vi "OutFlagJudge.vi"(8 "error in":errorcluster caption="错误输入", 11 "包装箱条码":string) -> (0 "error out":errorcluster caption="错误输出", 2 "Str":string, 3 "OK?":bool)   [LabVIEW 2013]
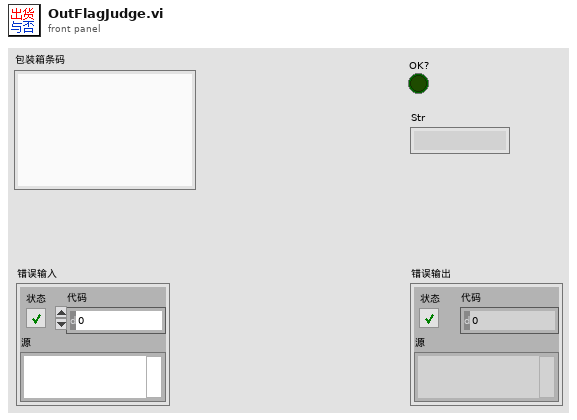
[diagram p1: front panel]
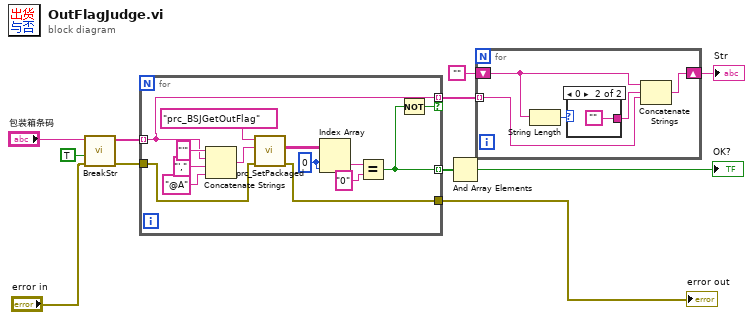
[diagram p0: block diagram]
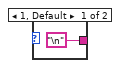
[diagram p2: hidden frame]
diagram:
  n1 = call "BreakStr.vi"("error in"="error in", "外购？"=TRUE, "StrIn"="包装箱条码") -> ("error out"=w9:errorcluster, "ArrayOut"=w10:string[])  [unwired: 7 in]
  n2 = for {
    tunnel: w10 -> [w16] mode=indexing
    tunnel: [w15] -> w5 mode=indexing
    tunnel: [w16] -> w8 mode=indexing if=w14
    tunnel: w9 -> [w13]
    tunnel: [w12] -> w1
    w19 = 0
    n3 = Concatenate Strings("'", w16, "',", "@A") -> (w22:string)
    n4 = call "prc_SetPackaged.vi"("error in"=w13, "string"=w22, "SQL query"="prc_BSJGetOutFlag") -> ("error out"=w12:errorcluster, "Array"=w20:string[][])  [unwired: 7 in]
    n5 = Index Array(array=w20, index (row)=w19, index (col)=w19) -> (element=w18:string)
    n6 = Equal?(x=w18, y="0") -> (x = y?=w15:bool)
    n7 = Not(x=w15) -> (.not. x?=w14:bool)
  }
  "error out" <- w1
  n8 = And Array Elements(Boolean array=w5) -> (logical AND=→"OK?":bool)
  n9 = for {
    tunnel: w8 -> [w27] mode=indexing
    shift-right: [w26] -> w6
    shift-left: "" -> [w28]
    n10 = String Length(string=w28) -> (length=w30:i32)
    n11 = case shown="0" w30 {
      tunnel: ["\n" ""] -> w29
      frame 1, Default {
      }
      frame 0 {
      }
    }
    n12 = Concatenate Strings(w28, w29, w27) -> (w26:string)
  }
  "Str" <- w6
